vi "lab1_0320Solovieva.vi"() -> ()   [LabVIEW 2020]
panel:
  out "If 1 triangle exists":string
  out "message":string
  in  "c":dbl
  in  "b":dbl
  in  "A":dbl
  out "S":dbl
  in  "2 sides and an angle":bool
  in  "Heron’s Formula":bool
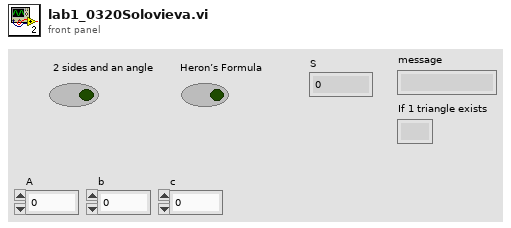
[diagram p1: front panel]
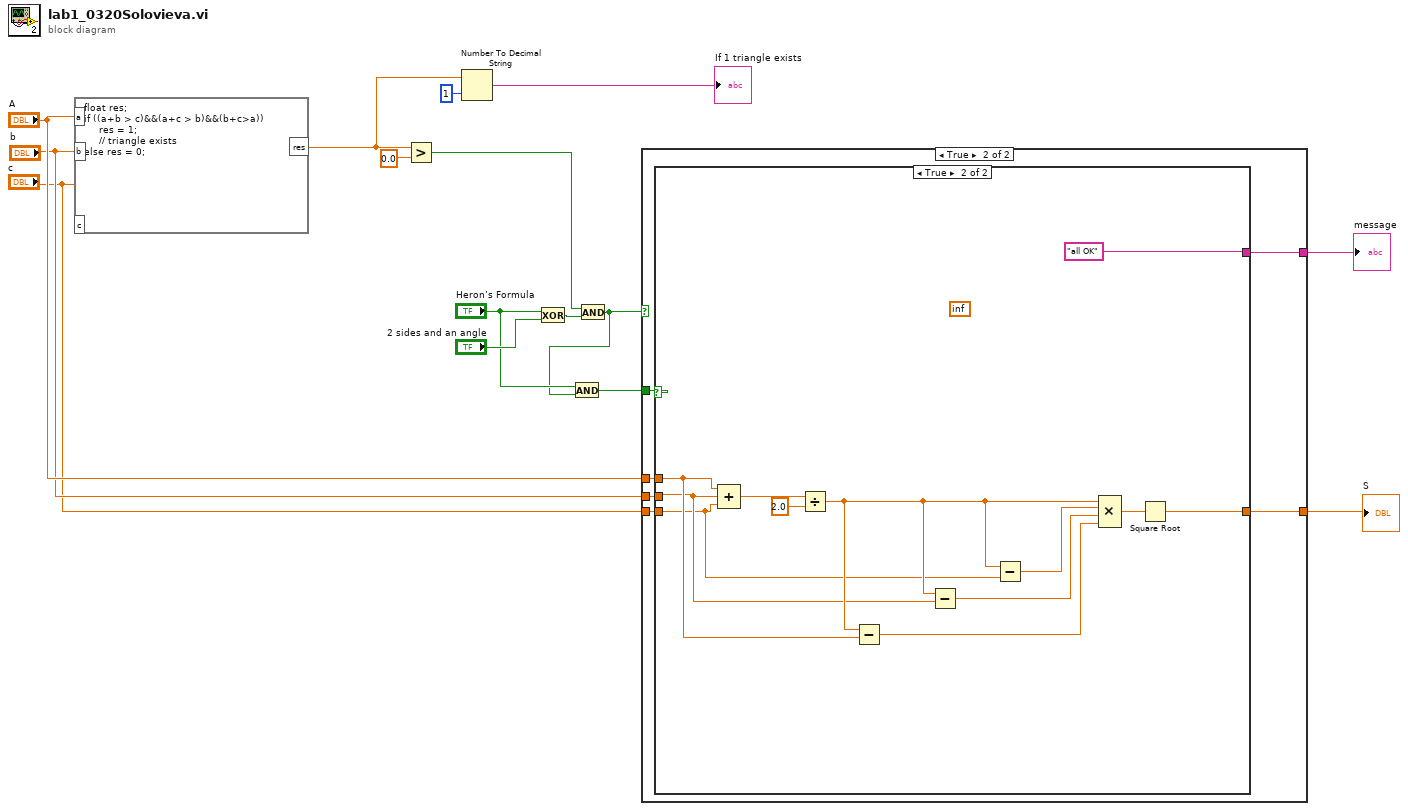
[diagram p0: block diagram]
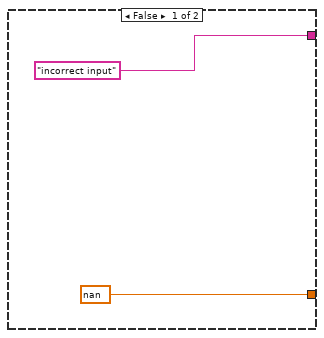
[diagram p2: hidden frame]
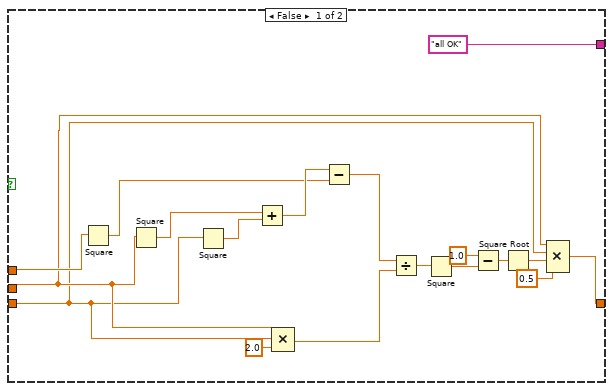
[diagram p3: hidden frame]
diagram:
  n1 = formula code="float res;\nif ((a+b > c)&&(a+c > b)&&(b+c>a))\n     res = 1;\n     // triangle exists\nelse res = 0;"("a"="A", "b"="b", "c"="c") -> ("res"=w3:dbl)
  n2 = Greater?(x=w3, y=0.0) -> (0:w4:bool)
  n3 = Number To Decimal String(number=w3, width (-)=i16 1) -> (decimal integer string=→"If 1 triangle exists":string)
  n4 = Exclusive Or(1:"2 sides and an angle", 2:"Heron’s Formula") -> (0:w11:bool)
  n5 = And(x=w4, y=w11) -> (x .and. y?=w10:bool)
  n6 = And(x="Heron’s Formula", y=w10) -> (x .and. y?=w13:bool)
  n7 = case shown="True" w10 {
    tunnel: w13 -> [_ w23]
    tunnel: "A" -> [_ w22]
    tunnel: "b" -> [_ w21]
    tunnel: "c" -> [_ w20]
    tunnel: [nan w19] -> w6
    tunnel: ["incorrect input" w18] -> w5
    frame False {
    }
    frame True {
      (unwired) inf
      n8 = case shown="True" w23 {
        tunnel: w22 -> [w28 w50]
        tunnel: w21 -> [w27 w49]
        tunnel: w20 -> [w25 w48]
        tunnel: [w26 w43] -> w19
        tunnel: ["all OK" "all OK"] -> w18
        frame False {
          n9 = Square(x=w28) -> (x^2=w38:dbl)
          n10 = Square(x=w27) -> (x^2=w41:dbl)
          n11 = Square(x=w25) -> (x^2=w40:dbl)
          n12 = Add(x=w40, y=w41) -> (x+y=w39:dbl)
          n13 = Compound Arithmetic op=MULTIPLY(w27, w25, 2.0 ("value")) -> (w35:dbl)
          n14 = Subtract(x=w39, y=w38) -> (x-y=w36:dbl)
          n15 = Divide(x=w36, y=w35) -> (x/y=w34:dbl)
          n16 = Square(x=w34) -> (x^2=w33:dbl)
          n17 = Subtract(x=1.0, y=w33) -> (x-y=w31:dbl)
          n18 = Square Root(x=w31) -> (sqrt(x)=w30:dbl)
          n19 = Compound Arithmetic op=MULTIPLY(w27, w25, w30, 0.5 ("value")) -> (w26:dbl)
        }
        frame True {
          n20 = Compound Arithmetic op=ADD(w50, w49, w48) -> (w53:dbl)
          n21 = Divide(x=w53, y=2.0) -> (x/y=w51:dbl)
          n22 = Subtract(x=w51, y=w50) -> (x-y=w45:dbl)
          n23 = Subtract(x=w51, y=w49) -> (x-y=w46:dbl)
          n24 = Subtract(x=w51, y=w48) -> (x-y=w47:dbl)
          n25 = Compound Arithmetic op=MULTIPLY(w51, w47, w46, w45) -> (w44:dbl)
          n26 = Square Root(x=w44) -> (sqrt(x)=w43:dbl)
        }
      }
    }
  }
  "S" <- w6
  "message" <- w5
